vi "Test Assertion Type for Pass If Error.vi"(8 "error in (no error)":errorcluster, 11 "Test Assertion Results in":refnum<class "Assertion Result Test.lvclass">) -> (0 "error out":errorcluster, 3 "Test Assertion Results out":refnum<class "Assertion Result Test.lvclass">)   [LabVIEW 2020, in "LUnit Tests.lvlib" / "Assertion Result Test.lvclass"]
uses:
  Assertion Result Test.lvclass
  Test Dummys/Test Case Test Double/Test Case Test Double.lvclass
  source/Framework/Result Types/Assertion Result/Public/TypeDefs/Assertion Type.ctl
  source/Framework/Result Types/Assertion Result/Assertion Result.lvlib
  <vilib>/Astemes/LUnit/Test Case.lvclass
panel:
  out "Assertion Type":T1
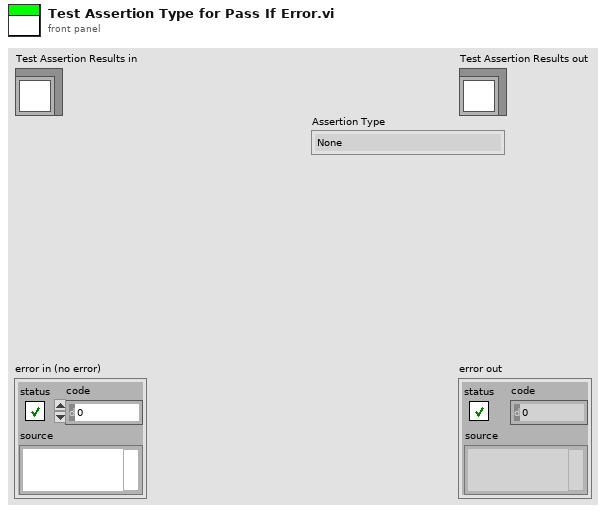
[diagram p1: front panel]
types:
  T1 = typedef "Assertion Result.lvlib/Assertion Type.ctl" = enum16{"None", "Pass", "Fail", "Skip", "Pass if Equal", "Fail if Equal", "Pass if Error", "Fail if Error", "Pass if", "Fail if"}
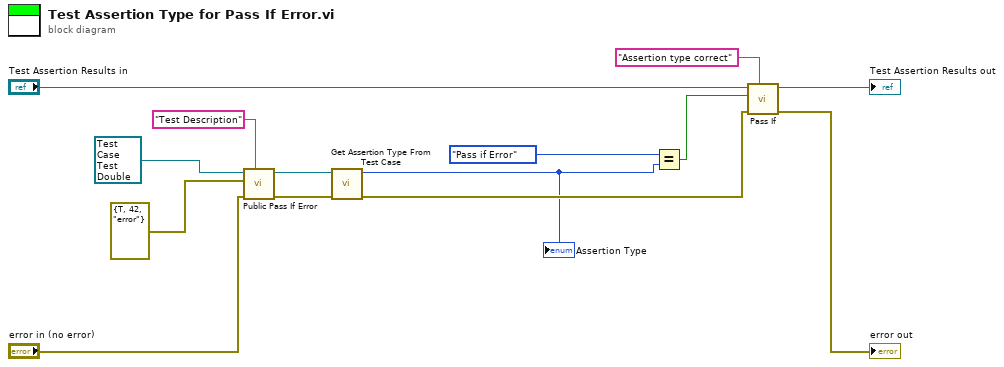
[diagram p0: block diagram]
diagram:
  n1 = call "Public Pass If Error.vi"("Description"="Test Description", "error in (no error)"="error in (no error)", "Assert error"=errorcluster {"status"=TRUE, "code"=42, "source"="error"}, "Test Case Test Double in"=refnum<class "Test Case Test Double.lvclass"> refnum ("Test Case Test Double.lvclass")) -> ("error out"=w11:errorcluster, "Test Case Test Double out"=w12:refnum<class "Test Case Test Double.lvclass">)  [unwired: 6 in]
  n2 = call "Get Assertion Type From Test Case.vi"("error in (no error)"=w11, "Test Case Test Double in"=w12) -> ("error out"=w2:errorcluster, "Assertion Type"=w1:T1)  [unwired: 8 in]
  "Assertion Type" <- w1
  n3 = Equal?(x=Assertion_Type."Pass if Error" ("Assertion Type"), y=w1) -> (x = y?=w5:bool)
  n4 = call <vilib>:"Pass If.vi"("Description"="Assertion type correct", "error in (no error)"=w2, "Pass?"=w5, "LUnit Test Case In"="Test Assertion Results in") -> ("error out"=→"error out":errorcluster, "LUnit Test Case Out"=→"Test Assertion Results out":refnum<class "Assertion Result Test.lvclass">)  [unwired: 6 in]
